vi "grSimTest.vi"(8 "error in (no error)":errorcluster, 10 "Reaplacement Tests":T3={"grSIM replacement"={"robots"=[], "ball"={"x"=0.0, "y"=0.0, "vx"=0.0, "vy"=0.0}}, "replace active"=FALSE, "TestParameters"={"Start"=FALSE, "V_sent"=4.0, "id"=0, "Samples"=0.0, "V_sample"=0.0, "delta"=0.0}, "Dest"=[4500.0, 3000.0], "V_desired"=4.0} {"Dest" format="%#_13g"}, 11 "Game in":refnum<class "Game.lvclass">) -> (0 "error out":errorcluster, 1 "grSim Test Replacement":bool, 2 "TestTeam":refnum<class "Ally.lvclass">, 3 "State":T2 {"progress" scale=0.0..100.0}, 4 "replaceBall":bool, 5 "velocityBreakState":T1)   [LabVIEW 2020, in "Game.lvclass"]
uses:
  Game.lvclass
  Controls/RobotModelReplacementTest.ctl
  Communication_class/Paths/grSim Packet Command UDP Test Folder/grSim/grSim RobotReplacement.ctl
  Communication_class/Paths/grSim Packet Command UDP Test Folder/grSim/grSim_BallReplacement.ctl
  Ally_class/Ally.lvclass
  Controls/RobotModelTestState.ctl
  VelocityPlanningTest/Controls/velocityBreakState.ctl
  Communication_class/Communication.lvclass
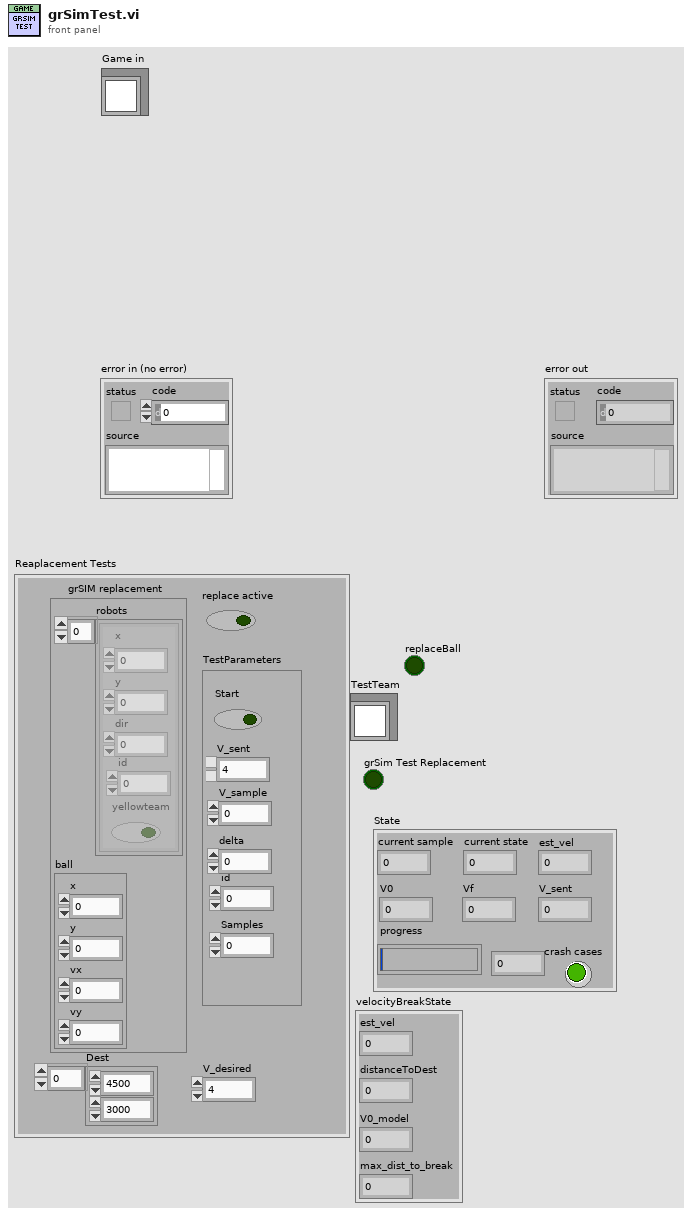
[diagram p1: front panel]
types:
  T1 = typedef "velocityBreakState.ctl" = cluster{"est_vel":dbl, "distanceToDest":dbl, "V0_model":dbl, "max_dist_to_break":dbl}
  T2 = typedef "RobotModelTestState.ctl" = cluster{"current sample":i32, "V0":dbl, "Vf":dbl, "progress":dbl, "current state":i32, "est_vel":dbl, "V_sent":dbl, "crash cases":bool}
  T3 = typedef "RobotModelReplacementTest.ctl" = cluster{"grSIM replacement":cluster{"robots":T4[], "ball":T5}, "replace active":bool, "TestParameters":cluster{"Start":bool, "V_sent":dbl, "id":i32, "Samples":dbl, "V_sample":dbl, "delta":dbl}, "Dest":dbl[], "V_desired":dbl}
  T4 = typedef "grSim RobotReplacement.ctl" = cluster{"x":dbl, "y":dbl, "dir":dbl, "yellowteam":bool, "id":u32}
  T5 = typedef "grSim_BallReplacement.ctl" = cluster{"x":dbl, "y":dbl, "vx":dbl, "vy":dbl}
  T6 = cluster{"Start":bool, "V_sent":dbl, "id":i32, "Samples":dbl, "V_sample":dbl, "delta":dbl}
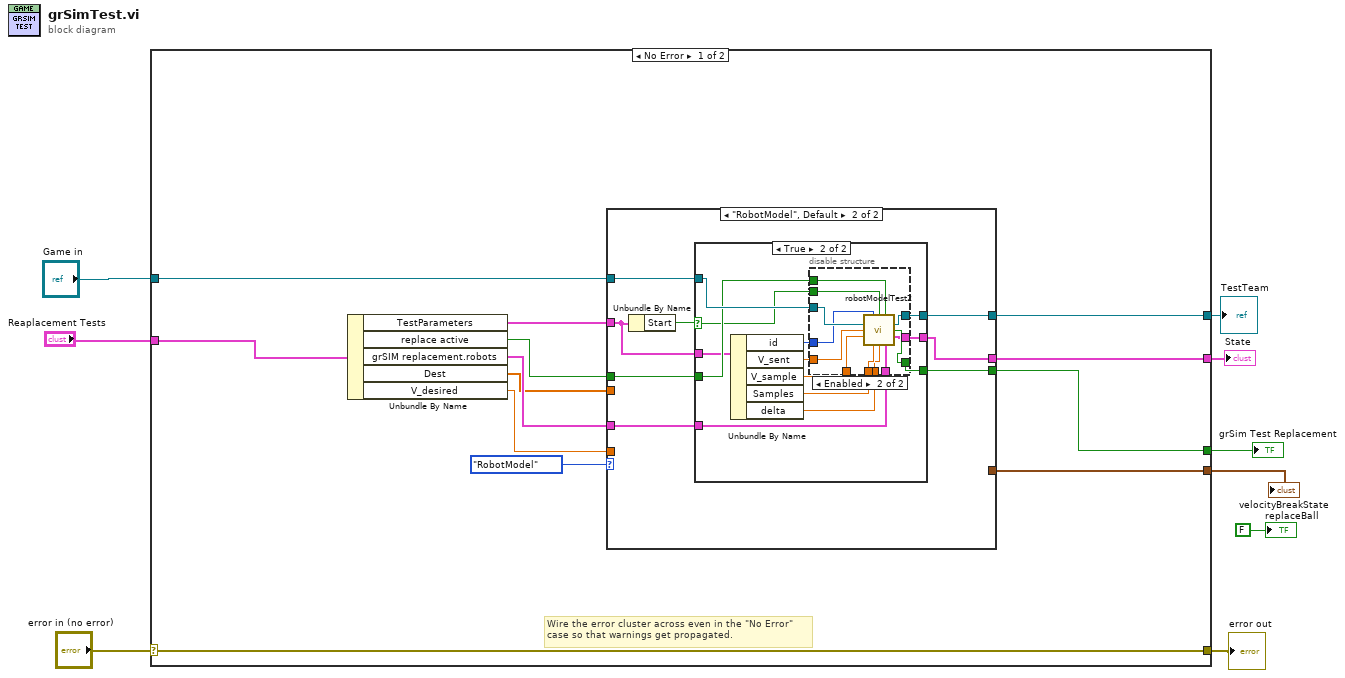
[diagram p0: block diagram]
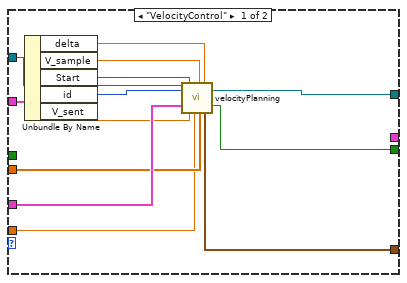
[diagram p2: hidden frame]
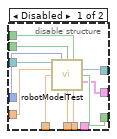
[diagram p4: hidden frame]
diagram:
  n1 = case shown="No Error" "error in (no error)" {
    selector: "error in (no error)" -> [w22 w81]
    tunnel: [w22 w81] -> w8
    tunnel: "Game in" -> [w18 _]
    tunnel: "Reaplacement Tests" -> [w19 _]
    tunnel: [w16 _] -> w5
    tunnel: [w17 _] -> w4
    tunnel: [w13 _] -> w3
    tunnel: [w12 _] -> w1
    frame No Error {
      # "Wire the error cluster across even in the \"No Error\"\ncase so that warnings get propagated."
      n2 = Unbundle By Name(w19) -> ("TestParameters"=w21:T6, "replace active"=w20:bool, "grSIM replacement.robots"=w15:T4[], "Dest"=w11:dbl[], "V_desired"=w10:dbl)
      n3 = case shown="\"RobotModel\", Default" enum16{"VelocityControl", "RobotModel"}."RobotModel" {
        tunnel: w21 -> [w34 w42]
        tunnel: w20 -> [_ w41]
        tunnel: w18 -> [w33 w40]
        tunnel: [w32 w39] -> w17
        tunnel: [w31 w38] -> w16
        tunnel: [_ w37] -> w13
        tunnel: w15 -> [w35 w36]
        tunnel: [w27 _] -> w12
        tunnel: w11 -> [w24 _]
        tunnel: w10 -> [w23 _]
        frame "VelocityControl" {
          n4 = Unbundle By Name(w34) -> ("delta"=w26:dbl, "V_sample"=w25:dbl, "Start"=w29:bool, "id"=w30:i32, "V_sent"=w28:dbl)
          n5 = call "velocityPlanning.vi"("Game in"=w33, "id"=w30, "robots"=w35, "start"=w29, "V_sent"=w28, "v_desired"=w23, "v_sample"=w25, "Dest"=w24, "delta"=w26) -> ("velocityBreakState"=w27:T1, "TestTeam"=w32:refnum<class "Ally.lvclass">, "replace"=w31:bool)  [unwired: 6 in, 2 out]
        }
        frame "RobotModel", Default {
          n6 = Unbundle By Name(w42) -> ("Start"=w43:bool)
          n7 = case shown="True" w43 {
            selector: w43 -> [_ w52]
            tunnel: w41 -> [w44 w56]
            tunnel: w40 -> [_ w57]
            tunnel: w42 -> [_ w55]
            tunnel: [_ w54] -> w39
            tunnel: [w44 w53] -> w38
            tunnel: [_ w46] -> w37
            tunnel: w36 -> [_ w45]
            frame False {
            }
            frame True {
              n8 = Unbundle By Name(w55) -> ("id"=w51:i32, "V_sent"=w50:dbl, "V_sample"=w49:dbl, "Samples"=w47:dbl, "delta"=w48:dbl)
              n9 = disable-structure shown="Enabled" {
                disable-tunnel: w57 -> [w68 w80]
                disable-tunnel: w56 -> [w67 w77]
                disable-tunnel: [w66 w71] -> w54
                disable-tunnel: [w65 w72] -> w53
                disable-tunnel: w52 -> [w64 w78]
                disable-tunnel: w51 -> [w63 w79]
                disable-tunnel: w50 -> [w62 w76]
                disable-tunnel: w49 -> [w61 w75]
                disable-tunnel: w48 -> [w60 w73]
                disable-tunnel: w47 -> [w59 w74]
                disable-tunnel: [w58 w70] -> w46
                disable-tunnel: w45 -> [_ w69]
                frame Disabled {
                  n10 = call "robotModelTest.vi"("Game in"=w68, "id"=w63, "Start"=w64, "replace active"=w67, "V_sent"=w62, "V_sample"=w61, "Samples"=w59, "delta"=w60) -> ("TestTeam"=w66:refnum<class "Ally.lvclass">, "Replace"=w65:bool, "State"=w58:T2)  [unwired: 3 in, 2 out]
                }
                frame Enabled {
                  n11 = call "robotModelTest2.vi"("id"=w79, "Start"=w78, "replace active"=w77, "Game in"=w80, "V_sent"=w76, "V_sample"=w75, "Samples"=w74, "delta"=w73, "grSIM replacement.robots"=w69) -> ("TestTeam"=w71:refnum<class "Ally.lvclass">, "Replace"=w72:bool, "State"=w70:T2)  [unwired: 2 in, 2 out]
                }
              }
            }
          }
        }
      }
    }
    frame Error {
    }
  }
  "error out" <- w8
  "grSim Test Replacement" <- w5
  "TestTeam" <- w4
  "State" <- w3
  "velocityBreakState" <- w1
  "replaceBall" <- FALSE ("replaceBall")
